vi "Task Type.vi"(11 "DataLogger in":refnum<class "DataLogger.lvclass">) -> (2 "Task Type":string)   [LabVIEW 2020, in "VolatusData.lvlib" / "DataLogger.lvclass"]
uses:
  DataLogger.lvclass
  DataLogger.lvclass/DataLogger.ctl
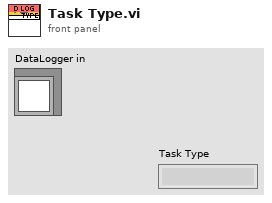
[diagram p1: front panel]
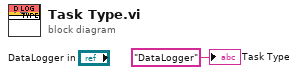
[diagram p0: block diagram]
diagram:
  "Task Type" <- "DataLogger" ("Task Type")
